vi "Dual Hall.vi"() -> ()   [LabVIEW 2015]
uses:
  <vilib>/DAQmx/read.llb/DAQmx Read (Analog 2D DBL NChan NSamp).vi
  <vilib>/DAQmx/create/channels.llb/DAQmx Create Channel (AI-Voltage-Basic).vi
  <vilib>/DAQmx/configure/timing.llb/DAQmx Timing (Sample Clock).vi
  <vilib>/DAQmx/miscellaneous.llb/DAQmx Fill In Error Info.vi
  <vilib>/Utility/file.llb/Write Delimited Spreadsheet (DBL).vi
  <vilib>/Analysis/NI_AALBase.lvlib
panel:
  in  "Log Btn":bool
  in  "Averages":u16=100
  in  "Log File":path=path "C:/Whiskeroscope.txt"
  out "XY Graph":cluster{"X":dbl, "Y":dbl}[](graph)
  out "Distance":dbl format="%6.3f"
  out "Force":dbl format="%6.3f"
  in  "Set Ref Btn":bool
  out "Offset 2":dbl format="%.2f"
  out "Offset 1":dbl format="%.2f"
  in  "Mean 2":dbl=2.4
  in  "Mean 1":dbl=2.55
  out "Amplitude":dbl[][](graph)
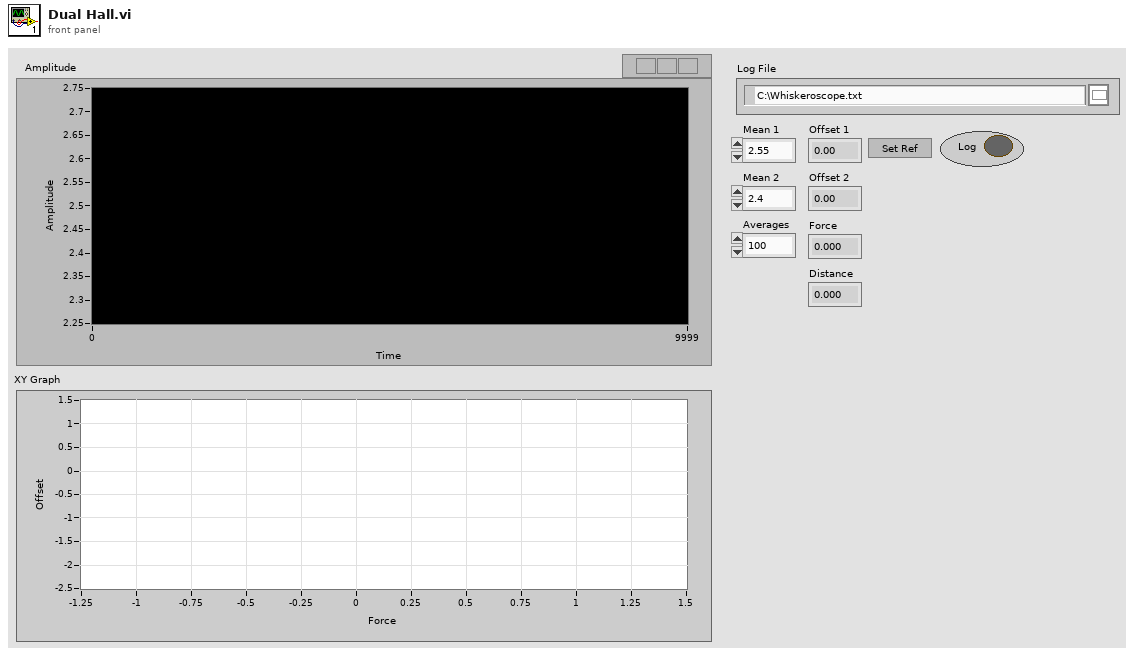
[diagram p1: front panel]
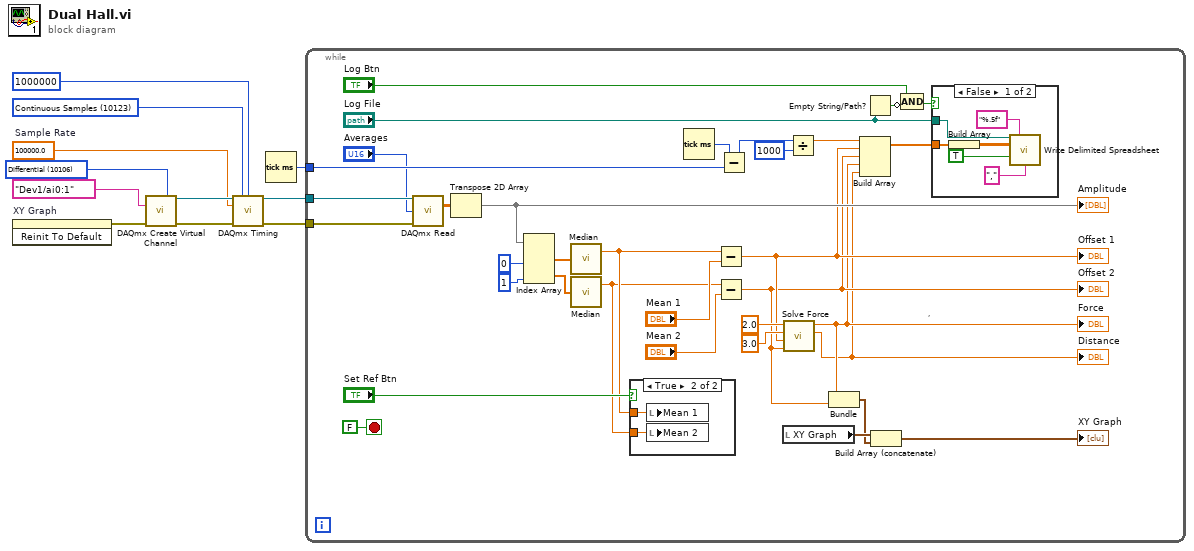
[diagram p0: block diagram]
diagram:
  w6 = 100000.0  # Sample Rate
  w5 = 10123 items=["Finite Samples"=10178, "Continuous Samples"=10123, "Hardware Timed Single Point"=12522] ("sample mode")
  w11 = 10106 items=["default"=-1, "RSE"=10083, "NRSE"=10078, "Differential"=10106, "Pseudodifferential"=12529] ("input terminal configuration")
  n1 = invoke on="XY Graph" class="XYGraph (strict)" method="Reinit To Default"() -> (error out=w2:errorcluster)  [unwired: 3 in, 2 out]
  n2 = call-poly <vilib>:"DAQmx Create Virtual Channel.vi"("input terminal configuration"=w11, "physical channels"=tag "Dev1/ai0:1", "error in"=w2) -> ("task out"=w10:refnum<k21>, "error out"=w9:errorcluster)  [unwired: 11 in]
  n3 = call-poly <vilib>:"DAQmx Timing.vi"("task/channels in"=w10, "sample mode"=w5, "samples per channel"=1000000, "rate"=w6, "error in"=w9) -> ("task out"=w8:refnum<k21>, "error out"=w7:errorcluster)  [unwired: 9 in]
  n4 = Tick Count (ms)() -> (millisecond timer value=w1:u32)
  n5 = while {
    tunnel: w8 -> [w45]
    tunnel: w7 -> [w44]
    tunnel: w1 -> [w19]
    stop <- FALSE stop-if-true
    # ","
    n6 = call-poly <vilib>:"DAQmx Read.vi"("task/channels in"=w45, "number of samples per channel"="Averages", "error in"=w44) -> ("data"=w42:dbl[][])  [unwired: 10 in, 2 out]
    n7 = Transpose 2D Array(2D array=w42) -> (transposed array=w41:dbl[][])
    "Amplitude" <- w41
    n8 = Index Array(array=w41, index (col) #1=0 ("index (row)"), index (col) #2=1 ("index (row)")) -> (element #1=w39:dbl[], element #2=w36:dbl[])  [unwired: 2 in]
    n9 = call <vilib>:"Median.vi"("X"=w39) -> ("median"=w37:dbl)  [unwired: 1 out]
    n10 = call <vilib>:"Median.vi"("X"=w36) -> ("median"=w35:dbl)  [unwired: 1 out]
    n11 = case shown="True" "Set Ref Btn" {
      tunnel: w37 -> [_ w53]
      tunnel: w35 -> [_ w52]
      frame False {
      }
      frame True {
        n12 = local write "Mean 1"(w53) -> ()
        n13 = local write "Mean 2"(w52) -> ()
      }
    }
    n14 = Tick Count (ms)() -> (millisecond timer value=w20:u32)
    n15 = Subtract(x=w37, y="Mean 1") -> (x-y=w26:dbl)
    "Offset 1" <- w26
    n16 = Subtract(x=w35, y="Mean 2") -> (x-y=w25:dbl)
    "Offset 2" <- w25
    n17 = Subtract(x=w20, y=w19) -> (x-y=w18:u32)
    n18 = local read "XY Graph"() -> (w29:cluster{"X":dbl, "Y":dbl}[])
    n19 = call "Solve Force.vi"("y2"=w25, "y1"=w26, "x2"=3.0 ("x1"), "x1"=2.0) -> ("D"=w23:dbl, "P"=w24:dbl)  [unwired: 6 in]
    "Force" <- w24
    "Distance" <- w23
    n20 = Divide(x=w18, y=u32 1000) -> (x/y=w17:dbl)
    n21 = Bundle("P"=w24, w25) -> (w27:cluster{"P":dbl, dbl})  [unwired: 1 in]
    n22 = Build Array(w17, w26, w25, w24, w23) -> (w22:dbl[])
    n23 = Empty String/Path?(string/path="Log File") -> (empty?=w14:bool)
    n24 = Build Array (concatenate)(w29, w27) -> (→"XY Graph":cluster{"P":dbl, "Y":dbl}[])
    n25 = Compound Arithmetic op=AND("Log Btn", invert w14) -> (w12:bool)
    n26 = case shown="False" w12 {
      tunnel: w22 -> [w51 _]
      tunnel: "Log File" -> [w48 _]
      frame False {
        n27 = Build Array(w51) -> (w50:dbl[][])
        n28 = call-poly <vilib>:"Write Delimited Spreadsheet.vi"("file path (dialog if empty)"=w48, "format (%.3f)"="%.5f", "2D data"=w50, "append to file? (F)"=TRUE, "delimiter (\\t)"="," ("delimiter (\\t)")) -> ()  [unwired: 9 in, 2 out]
      }
      frame True {
      }
    }
  }
